vi "Prepare Queue.vi"(8 "Error In":errorcluster) -> (0 "Error Out":errorcluster, 3 "TDMS Log Queue":refnum<queue>)   [LabVIEW 2014, in "TDMS Logger.lvlib" / "TDMS Logger.lvclass"]
uses:
  TDMS Logger.lvclass
  _Typedefs/Log Message.ctl
  _Typedefs/Log Action.ctl
  _Typedefs/Data Type.ctl
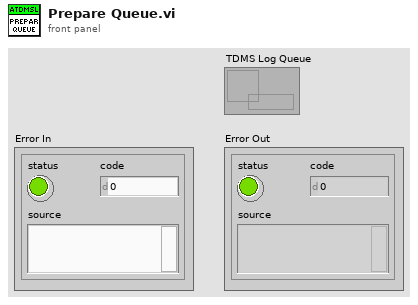
[diagram p1: front panel]
types:
  T1 = typedef "TDMS Logger.lvlib/TDMS Logger.lvclass/Log Action.ctl" = enum16{"Handle Old Files", "Status Update", "Stop", "Log Data", "Initialize"}
  T2 = typedef "TDMS Logger.lvlib/TDMS Logger.lvclass/Log Message.ctl" = cluster{"Log Action":T1, "Variant":variant, "Data Type":T3, "Group Name":string, "Channels Names":string[]}
  T3 = typedef "TDMS Logger.lvlib/TDMS Logger.lvclass/Data Type.ctl" = enum16{"I16", "I8", "String", "U16", "U8", "Waveform", "Double", "Single"}
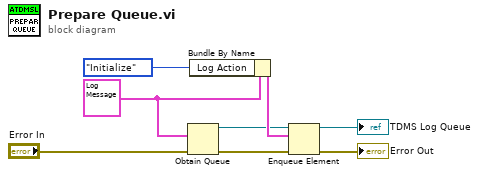
[diagram p0: block diagram]
diagram:
  w6 = T2 {"Log Action"=enum."Stop", "Variant"=variant, "Data Type"=enum."String", "Group Name"="", "Channels Names"=[]}
  n1 = Obtain Queue(element data type=w6, error in (no error)="Error In") -> (queue out=w2:refnum<queue>, error out=w3:errorcluster)  [unwired: 3 in, 1 out]
  n2 = Bundle By Name(cluster=w6, "Log Action"=Log_Action."Initialize") -> (w7:T2)
  n3 = Enqueue Element(queue=w2, element=w7, error in (no error)=w3) -> (queue out=→"TDMS Log Queue":refnum<queue>, error out=→"Error Out":errorcluster)  [unwired: 1 in, 1 out]
